vi "tsc_Search Ring.vi"(10 "Values":string[](array[string]), 11 "Search Item":string) -> (3 "Index":u16)   [LabVIEW 2021]
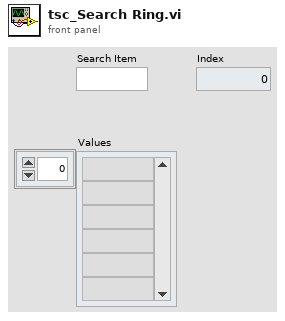
[diagram p1: front panel]
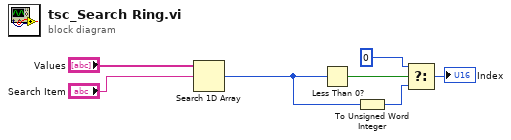
[diagram p0: block diagram]
diagram:
  n1 = Search 1D Array(1D array="Values", element="Search Item") -> (index of element=w2:i32)  [unwired: 1 in]
  n2 = Less Than 0?(x=w2) -> (x < 0?=w4:bool)
  n3 = To Unsigned Word Integer(number=w2) -> (unsigned 16bit integer=w1:u16)
  n4 = Select(t=u16 0, s=w4, f=w1) -> (s? t:f=→"Index":u16)
